vi "CB Remote Sense Test_v2.vi"(8 "error in (no error)":errorcluster, 11 "ControlBoard VISA":refnum<visa-resource-name>="ControlBoard") -> (0 "error out":errorcluster, 1 "Pass?":bool, 2 "Message OUT":string, 3 "Control Board OUT":refnum<visa-resource-name>)   [LabVIEW 2022 SP3]
panel:
  out "MSE Array":dbl[](array[numeric])
  out "Voltage Readings":dbl[][](array[numeric])
  in  "Message IN":string
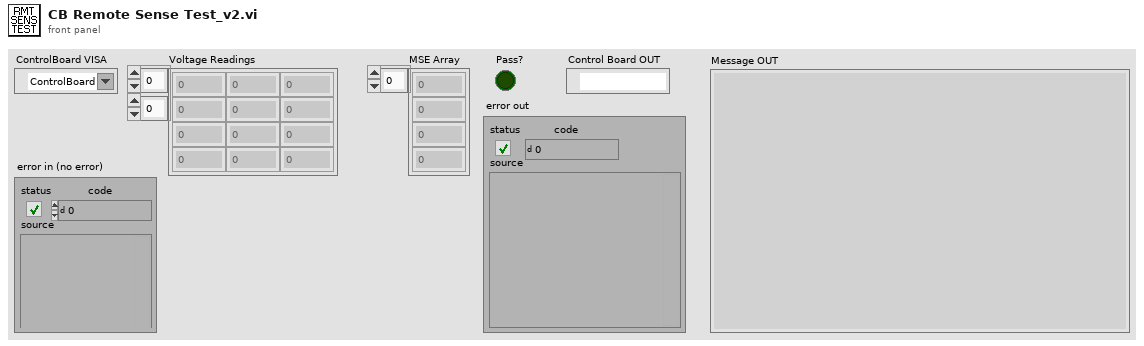
[diagram p1: front panel]
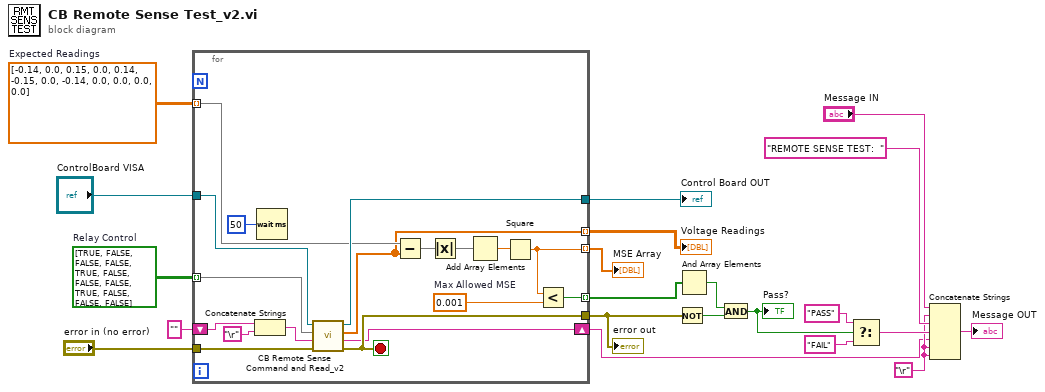
[diagram p0: block diagram]
diagram:
  w1 = dbl[][] [[-0.14, 0.0, 0.15], [0.0, 0.14, -0.15], [0.0, -0.14, 0.0], [0.0, 0.0, 0.0]]  # Expected Readings
  w9 = "\r"
  w19 = bool[][] [[TRUE, FALSE, FALSE], [FALSE, TRUE, FALSE], [FALSE, FALSE, TRUE], [FALSE, FALSE, FALSE]]  # Relay Control
  n1 = for {
    tunnel: [w37] -> w2
    tunnel: [w39] -> w21
    tunnel: "error in (no error)" -> [w38]
    tunnel: w1 -> [w34] mode=indexing
    tunnel: [w31] -> w20 mode=indexing
    tunnel: w19 -> [w30] mode=indexing
    tunnel: [w29] -> w16 mode=indexing
    tunnel: [w28] -> w15 mode=indexing
    shift-right: [w27] -> w7
    shift-left: "" -> [w26]
    tunnel: "ControlBoard VISA" -> [w22]
    stop <- w37 stop-if-true
    w32 = 0.001  # Max Allowed MSE
    n2 = Concatenate Strings(w26, "\r") -> (w25:string)
    n3 = Wait (ms)(milliseconds to wait=u32 50) -> ()  [unwired: 1 out]
    n4 = call "CB Remote Sense Command and Read_v2.vi"("error in (no error)"=w38, "Message IN"=w25, "Relay Control"=w30, "ControlBoard VISA"=w22) -> ("error out"=w37:errorcluster, "Message OUT"=w27:string, "Voltage Array"=w29:dbl[], "Control Board OUT"=w39:refnum<visa-resource-name>)  [unwired: 4 in]
    n5 = Subtract(x=w34, y=w29) -> (x-y=w36:dbl[])
    n6 = Absolute Value(x=w36) -> (abs(x)=w35:dbl[])
    n7 = Add Array Elements(numeric array=w35) -> (sum=w33:dbl)
    n8 = Square(x=w33) -> (x^2=w28:dbl)
    n9 = Less?(x=w28, y=w32) -> (x < y?=w31:bool)
  }
  "error out" <- w2
  "Voltage Readings" <- w16
  "MSE Array" <- w15
  "Control Board OUT" <- w21
  n10 = Not(x=w2) -> (.not. x?=w17:bool)
  n11 = And Array Elements(Boolean array=w20) -> (logical AND=w18:bool)
  n12 = And(x=w18, y=w17) -> (x .and. y?=w8:bool)
  "Pass?" <- w8
  n13 = Select(t="PASS", s=w8, f="FAIL") -> (s? t:f=w13:string)
  n14 = Concatenate Strings("Message IN", w9, "REMOTE SENSE TEST:  ", w13, w7, w9, w9) -> (→"Message OUT":string)
